vi "DAY 2 part 3 (1).vi"() -> ()   [LabVIEW 2025]
panel:
  out "element 5":dbl
  in  "array 3":dbl[][](array[numeric])
  out "element 4":dbl
  in  "array 2":dbl[][](array[numeric])
  out "appended array 2":dbl[][](array[numeric])
  in  "element 3":dbl[][](array[numeric])
  out "appended array":dbl[](array[numeric])
  in  "element 2":dbl
  in  "element":dbl
  out "size(s)":i32
  in  "array":dbl[](array[numeric])
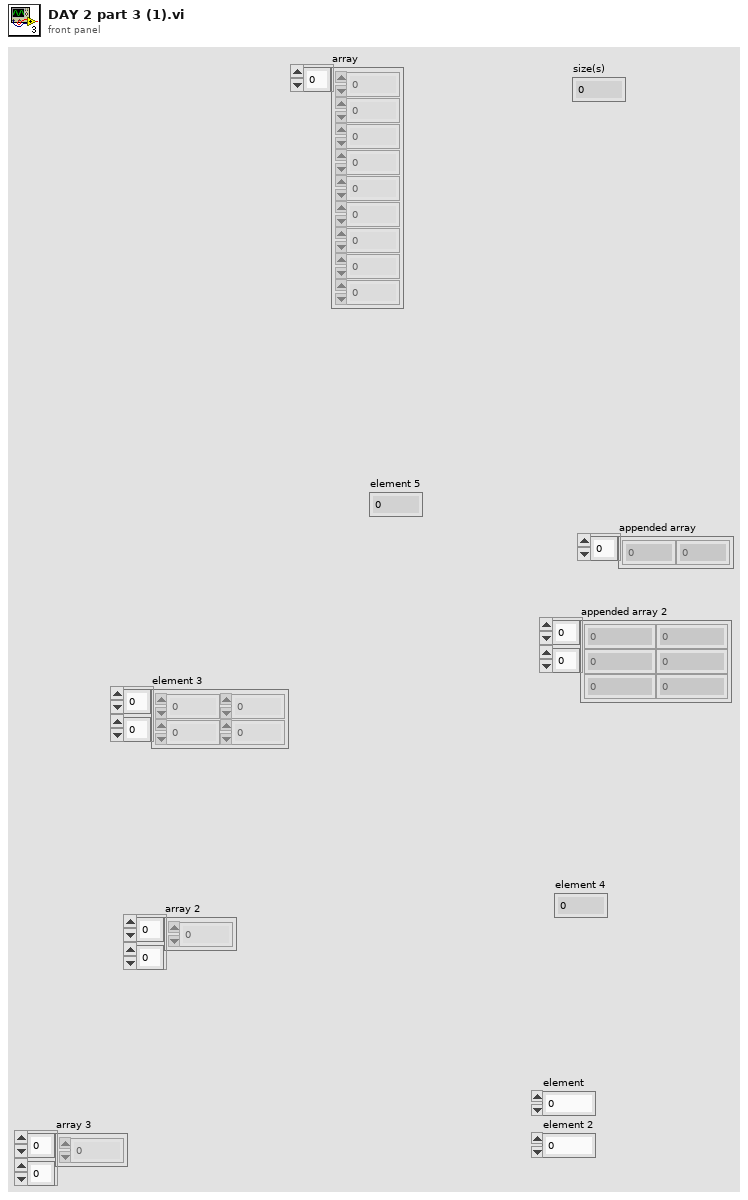
[diagram p1: front panel]
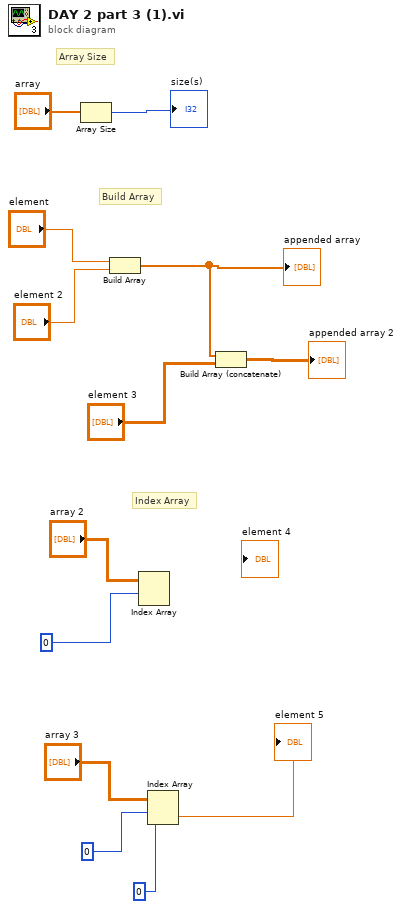
[diagram p0: block diagram]
diagram:
  # "Index Array"
  # "Build Array"
  # "Array Size"
  n1 = Array Size(array="array") -> (size(s)=→"size(s)":i32)
  n2 = Build Array("element", "element 2") -> (w9:dbl[])
  "appended array" <- w9
  n3 = Index Array(array="array 2", index (row)=0 ("index")) -> ()  [unwired: 1 in, 1 out]
  n4 = Index Array(array="array 3", index (row)=0, index (col)=0 ("disabled index (col)")) -> (element=→"element 5":dbl)
  n5 = Build Array (concatenate)(w9, "element 3") -> (→"appended array 2":dbl[][])
